vi "Get Available FPGA Components.vi"(8 "error in (no error)":errorcluster, 10 "Register Info":T3) -> (0 "error out":errorcluster, 3 "Bitfile Signature":string)   [LabVIEW 2012, in "AIT 429 System Explorer.lvlib"]
uses:
  <userlib>/_FPGA Interface Advanced Tools/FPGA Bitfile Utility/TypeDefs/Scalar Register Set.ctl
  <userlib>/_FPGA Interface Advanced Tools/FPGA Bitfile Utility/TypeDefs/Scalar Register.ctl
  AIT 429 System Explorer.lvlib
  <userlib>/_FPGA Interface Advanced Tools/FPGA Bitfile Utility/FPGA Bitfile Utility.lvlib
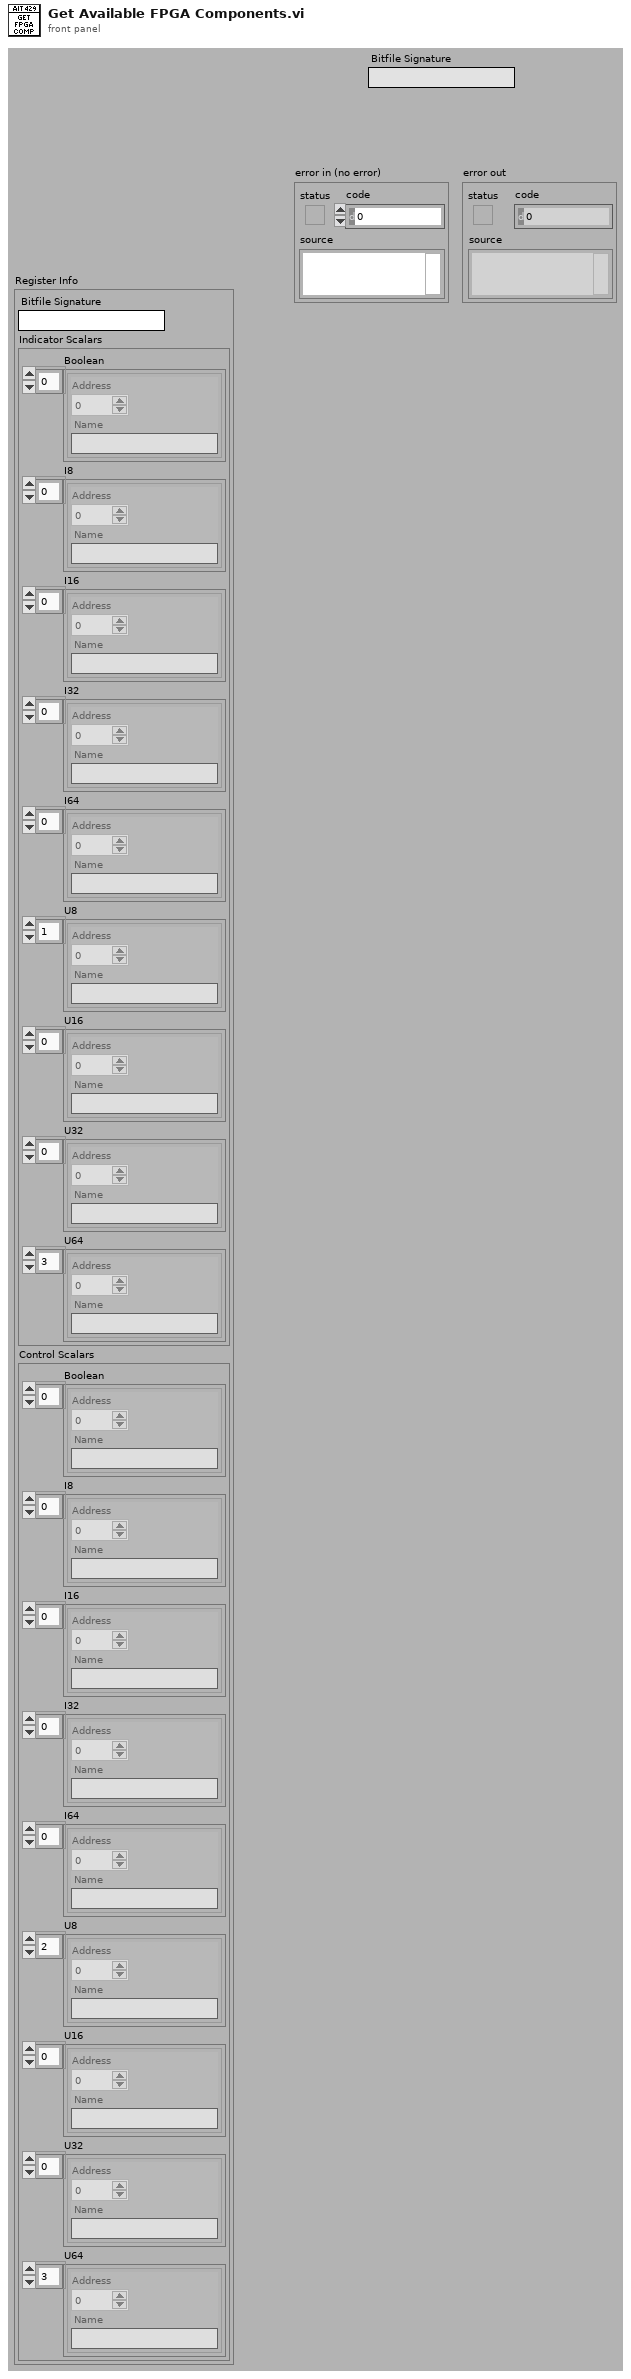
[diagram p1: front panel]
types:
  T1 = typedef "FPGA Bitfile Utility.lvlib/Scalar Register Set.ctl" = cluster{"Boolean":T2[], "I8":T2[], "I16":T2[], "I32":T2[], "I64":T2[], "U8":T2[], "U16":T2[], "U32":T2[], "U64":T2[]}
  T2 = typedef "FPGA Bitfile Utility.lvlib/Scalar Register.ctl" = cluster{"Address":u32, "Name":string}
  T3 = cluster{"Bitfile Signature":string, "Indicator Scalars":T1, "Control Scalars":T1}
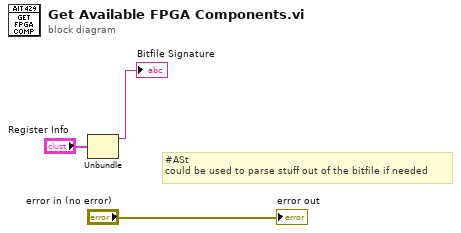
[diagram p0: block diagram]
diagram:
  # "#ASt\ncould be used to parse stuff out of the bitfile if needed"
  n1 = Unbundle("Register Info") -> ("Bitfile Signature"=→"Bitfile Signature":string)  [unwired: 2 out]
  "error out" <- "error in (no error)"
